vi "Get Run.vi"(8 "error in (no error)":errorcluster, 10 "index":i32, 11 "Schedule in":refnum<class "Schedule.lvclass">) -> (0 "error out":errorcluster, 1 "Repetitions":u32, 2 "Run Instance":refnum<class "Run Instance.lvclass">, 3 "Schedule out":refnum<class "Schedule.lvclass">)   [LabVIEW 2020, in "Run Utilities.lvlib" / "Schedule.lvclass"]
uses:
  Schedule.lvclass
  Run Instance/Run Instance.lvclass
  Schedule.lvclass/Schedule.ctl
  Cell/Schedule Cell.lvclass
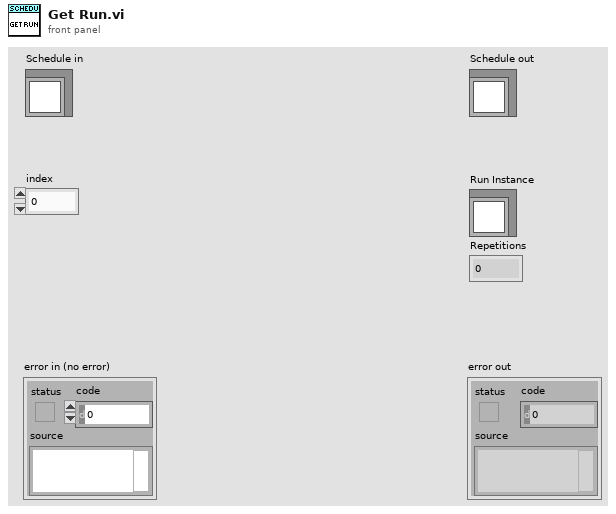
[diagram p1: front panel]
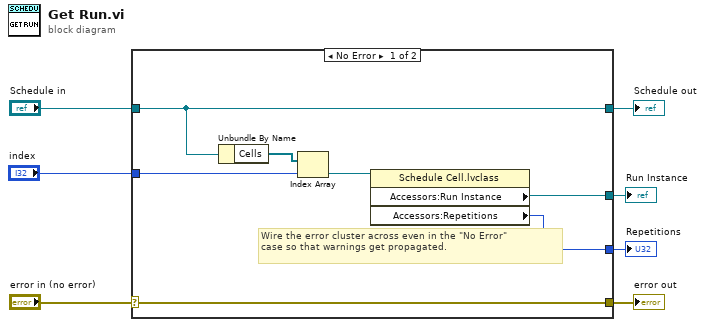
[diagram p0: block diagram]
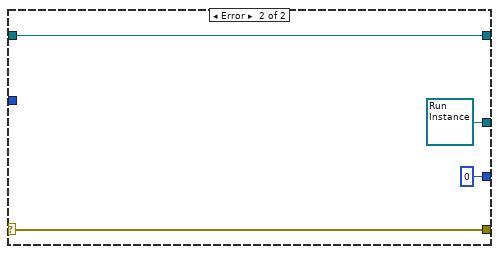
[diagram p2: hidden frame]
diagram:
  n1 = case shown="No Error" "error in (no error)" {
    selector: "error in (no error)" -> [w14 w18]
    tunnel: [w14 w18] -> w6
    tunnel: [w13 w17] -> w4
    tunnel: "Schedule in" -> [w13 w17]
    tunnel: "index" -> [w11 _]
    tunnel: [w9 refnum<class "Run Instance.lvclass"> refnum ("Run Instance")] -> w2
    tunnel: [w8 u32 0 ("Repetitions")] -> w1
    frame No Error {
      # "Wire the error cluster across even in the \"No Error\"\ncase so that warnings get propagated."
      n2 = Unbundle By Name(w13) -> ("Cells"=w12:refnum<class "Schedule Cell.lvclass">[])
      n3 = Index Array(array=w12, index=w11) -> (element=w10:refnum<class "Schedule Cell.lvclass">)
      n4 = property class="Schedule Cell.lvclass"(reference=w10) -> ("Accessors:Run Instance"=w9:refnum<class "Run Instance.lvclass">, "Accessors:Repetitions"=w8:u32)  [unwired: 1 in, 2 out]
    }
    frame Error {
    }
  }
  "error out" <- w6
  "Schedule out" <- w4
  "Run Instance" <- w2
  "Repetitions" <- w1
